vi "Detector GUI.vi"(9 "Standalone":bool=TRUE, 10 "Init Data":variant, 11 "Detector Name":string(combo)="PRIME") -> ()   [LabVIEW 2024]
uses:
  RIMAS Observation Config.ctl
  RIMAS Detector Server Config.ctl
  Detector Class/Detector enum Detector Integration Mode.ctl
  typedefs/CC enum Operation Mode.ctl
  Subsystems/SS typedef cluster Instrument Command Queue Data.ctl
  Subsystems/SS cluster Data Queue type.ctl
  RIMAS Detector Config.ctl
  Detector Class/Detector Image typedef cluster.ctl
  Detector Class/Detector Class.lvclass
  typedefs/CC cluster Observation.ctl
  Observation Queue/CC enum Observation Status.ctl
  Telescope/CC cluster Telescope Offsets.ctl
  typedefs/CC cluster Observation Dither Options.ctl
  typedefs/CC enum Dither Selection.ctl
  Detector Class/Detector cluster Files.ctl
  Detector Class/RIMAS Detector/RIMAS Detector.lvclass
  C:/Development/Prime-RIMAS/Detector/Detector Class/Detector Class.lvclass
  Detector Class/PRIME Detector/PRIME Detector.lvclass
  Detector Simulator/Detector Simulator.lvclass
  typedefs/CC cluster Alarm Data.ctl
  typedefs/CC cluster Exposure.ctl
  Detector Class/Detector Class.lvclass/Detector Class.ctl
  Subsystems/SS cluster New Image Data.ctl
  8cac10b2-9031-4085-930a-abf5b5c9cf51.vi
  Detector Class/Write Object Name.vi
panel:
  in  "Mode":T1
  in  "Tab Control":T2(tab)
  in  "Re-init":bool
  in  "Target Name":string
  out "Number Frames":i32
  in  "Integration Mode":T3
  in  "Integration Time":dbl=3.0 min=3.0 format="%_3g"
  in  "Image List":i32(listbox)
  out "Wait Message":string
  in  "send config":bool
  out "image":sgl[][](graph)
  in  "Get Image":bool
  out "Connected":bool
  in  "Reconnect":bool
  in  "FITS Detector Settings":T4
  in  "Frame Integration Time":dbl
  in  "Sim FITS File Path":path
  in  "Offsets":u16[][](array[numeric]) format="%04x"
  in  "FITS Data File Path":path
  in  "FITS hdr template1":path
  in  "FITS hdr template0":path
  in  "Detector Computer":T5={"Machine"="192.168.121.11", "Password"="", "FITS File Path"="", "Port"=44444, "Header Path"="", "Name"=""}
  in  "Show Log":bool
  in  "Clear Log":bool
  out "Messages":string
  in  "Close":bool
  # "seconds"
  # "Woring 4/8/2022 -- Always force CLOSE when intializing, then \nrestart the server."
  # "sec"
  # "sec"
  # "Seconds"
  # "Use \"Simulation\" if no detector"
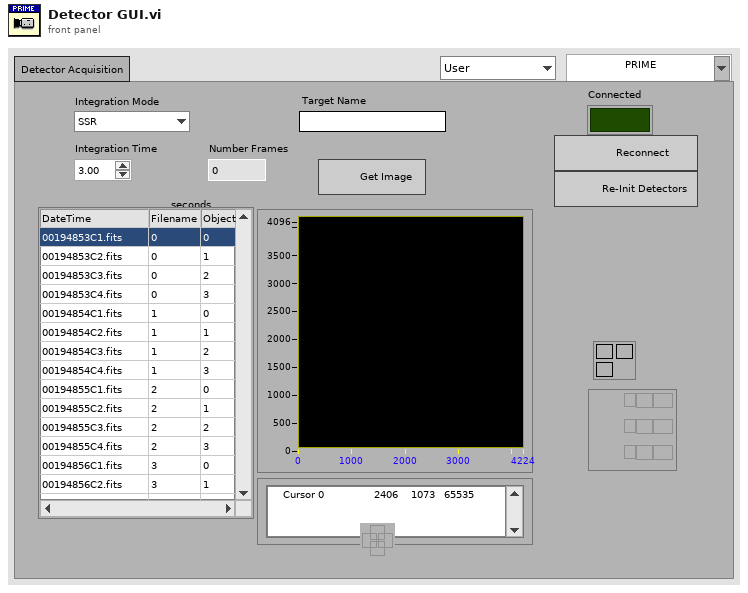
[diagram p1: front panel]
types:
  T1 = typedef "CC enum Operation Mode.ctl" = enum16{"User", "Engineering"}
  T2 = enum32{"Detector Acquisition", "Advanced Settings", "Settings", "Log", "Inputs"}
  T3 = typedef "Detector enum Detector Integration Mode.ctl" = enum16{"SSR", "CDS", "MEAN", "MEDIAN", "MODE", "MIIN", "MAX"}
  T4 = typedef "RIMAS Observation Config.ctl" = cluster{"Exp Time Short":dbl, "# of Frames":dbl, "Exp Time Long":dbl, "# of Groups":dbl, "Object Name":string, "Object":string, "Obs Type":string, "Image Type":string, "Observer":string, "Observer Affiliation":string}
  T5 = typedef "RIMAS Detector Server Config.ctl" = cluster{"Machine":string, "Password":string, "FITS File Path":string, "Port":u16, "Header Path":string, "Name":string}
  T6 = typedef "SS typedef cluster Instrument Command Queue Data.ctl" = cluster{"Cmd":string, "Parameters":variant}
  T7 = typedef "RIMAS Detector Config.ctl" = cluster{"Detector":u16, "Offsets":u16[][], "Detector Computer":T5, "FITS hdr template0":path, "FITS hdr template1":path, "FITS Data File Path":path, "FITS Detector Settings":T4, "Sim Folder":path, "Integration Mode":T3, "Integration Time":dbl, "Frame Int Time":dbl}
  T8 = typedef "Detector Class.lvclass/Detector Image typedef cluster.ctl" = cluster{"Image":sgl[][], "Frame number":i32, "Detector #":u16, "FITS file":path, "File size":i64}
  T9 = typedef "CC cluster Observation.ctl" = cluster{"Priority":i32, "ID":string, "Observer":string, "Obj Name":string, "Obj Type":string, "RA and DEC String":cluster{"RA":string, "DEC":string}, "Filter Wheel 1":string, "Filter Wheel 2":string, "Integration Time":dbl, "Observation Status":T10, "Offsets":T11, "Images":i32, "Dither Options":T12, "Comment 1":string, "Comment 2":string}
  T10 = typedef "CC enum Observation Status.ctl" = enum16{"Ready", "Running", "Done", "Error"}
  T11 = typedef "CC cluster Telescope Offsets.ctl" = cluster{"RA":dbl, "DEC":dbl, "ROT":dbl}
  T12 = typedef "CC cluster Observation Dither Options.ctl" = cluster{"Dither":T13, "Dither Radius":dbl, "Dither Points":i32, "Dither Phase":dbl}
  T13 = typedef "CC enum Dither Selection.ctl" = enum16{"None", "Circle", "Random"}
  T14 = typedef "Detector Class.lvclass/Detector cluster Files.ctl" = cluster{"Time":timestamp, "Files":path[][], "Total Frames":i32}
  T15 = cluster{"state":refnum<user-event>, "cmd q":refnum<queue>, "Cmd":T6, "Data Q":refnum<queue>, "error":errorcluster, "next poll":timestamp, "ch names":string[][], "Detector Config":T7, "images cnt":i32, "Images":T8[], "Name":string, "script q":refnum<queue>, "New Images":T8[], "FITS settings":T4, "Detector ref":refnum<class "Detector Class.lvclass">, "Connected":bool, "Observation":T9, "Raw Files":T14}
  T16 = enum8{"Enabled", "Disabled", "Disabled and Grayed Out"}
  T17 = typedef "CC cluster Alarm Data.ctl" = cluster{"Measured Value":dbl, "Alarm Low":dbl, "Alarm High":dbl, "Message":string, "Source":string}
  T18 = typedef "SS cluster Data Queue type.ctl" = cluster{"Source":string, "Type":string, "Data":variant}
  T19 = typedef "CC cluster Exposure.ctl" = cluster{"Mode":T3, "Integration Time":dbl, "Name":string, "Images":i32}
  T20 = typedef "SS cluster New Image Data.ctl" = cluster{"Frame number":i32, "Detector #":u16, "FITS file":path, "File size":i64}
  T21 = typedef "CC Current Status.ctl" = cluster{"Target":string, "Filter 1":string, "Filter 2":string}
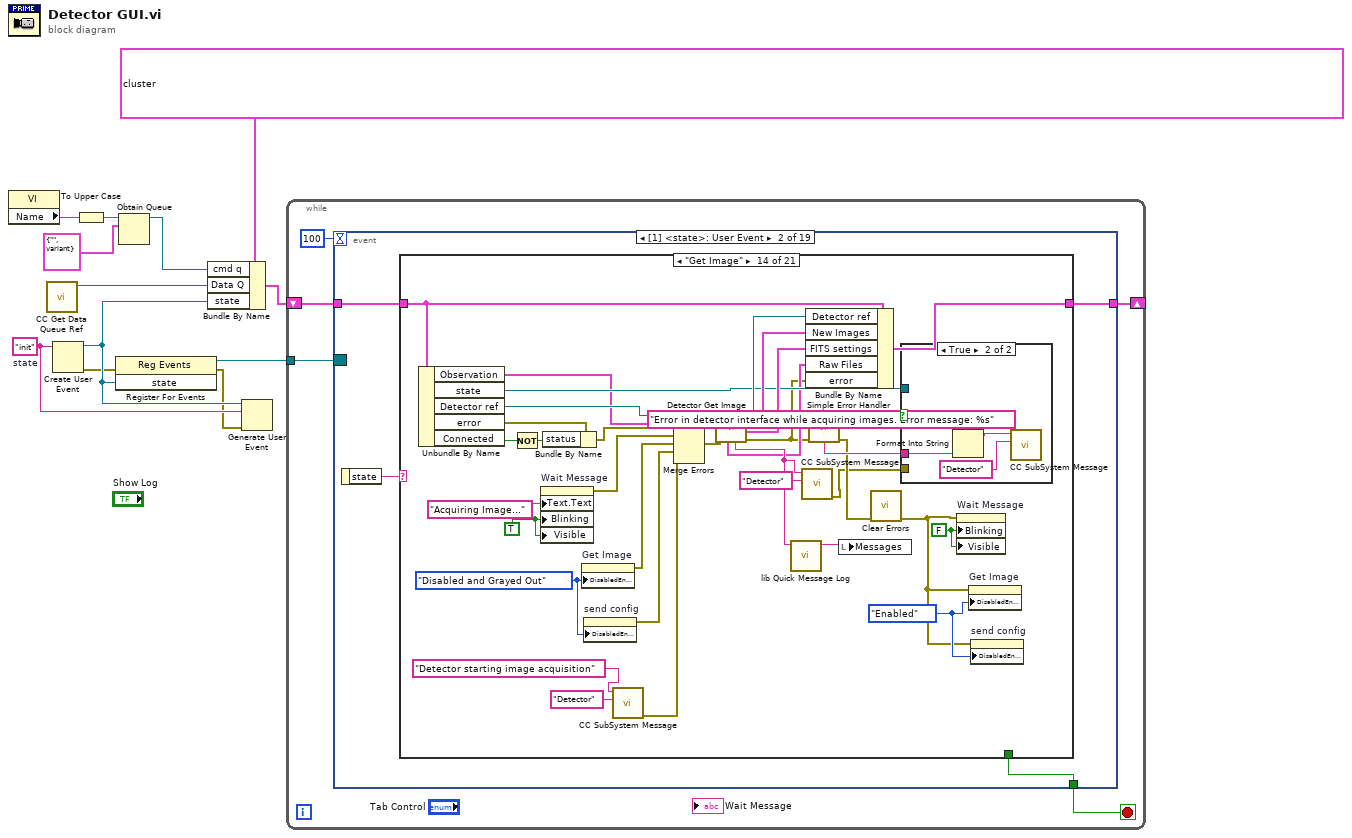
[diagram p0: block diagram]
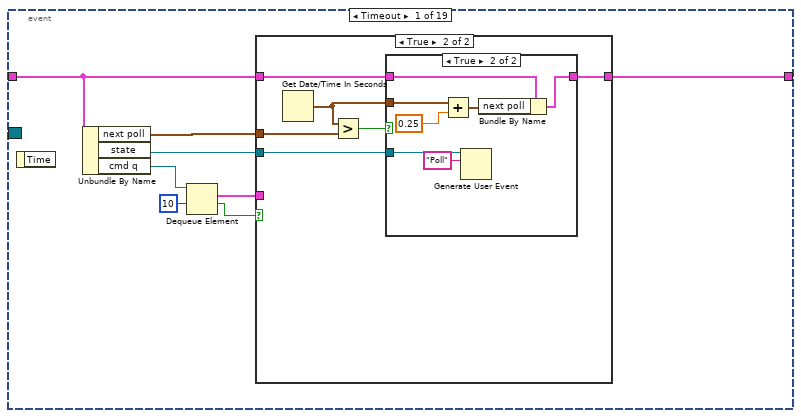
[diagram p2: hidden frame]
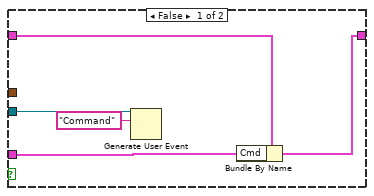
[diagram p3: hidden frame]
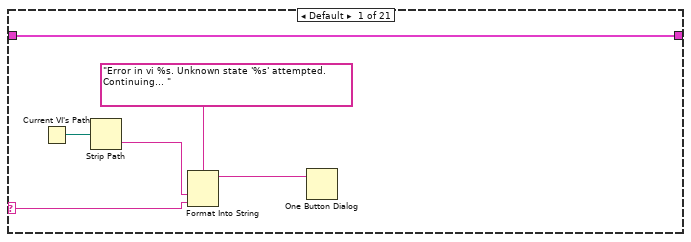
[diagram p5: hidden frame]
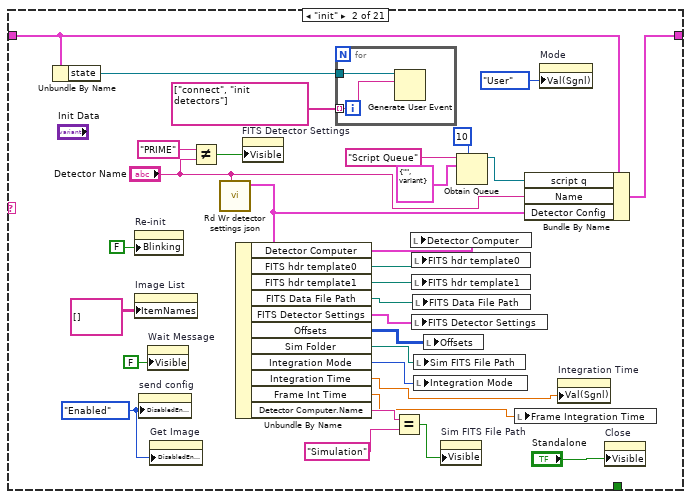
[diagram p6: hidden frame]
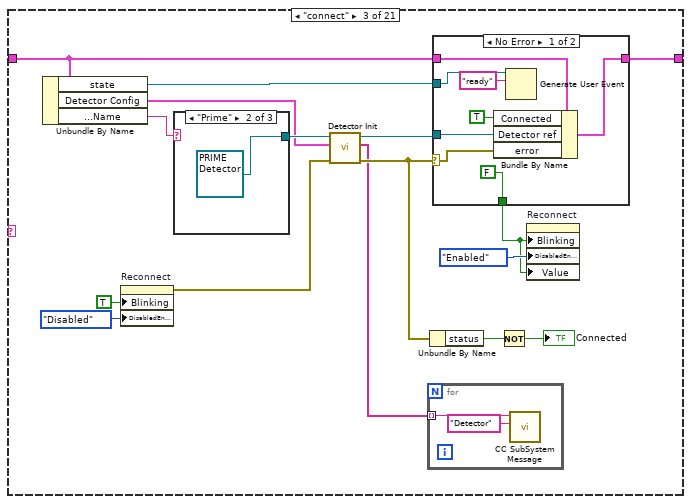
[diagram p7: hidden frame]
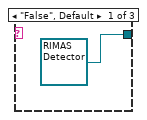
[diagram p8: hidden frame]
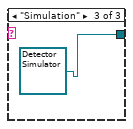
[diagram p9: hidden frame]
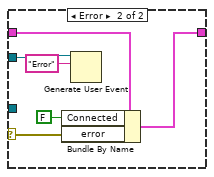
[diagram p10: hidden frame]
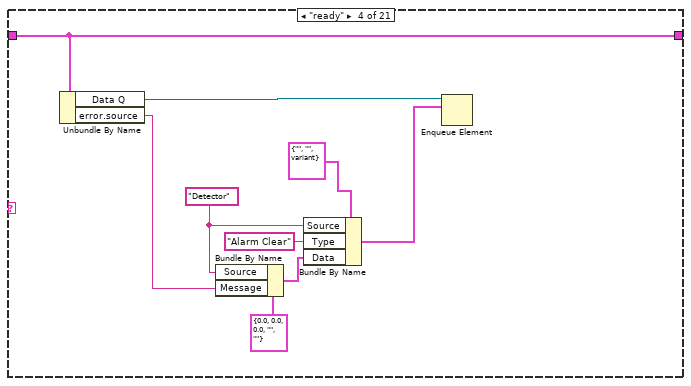
[diagram p11: hidden frame]
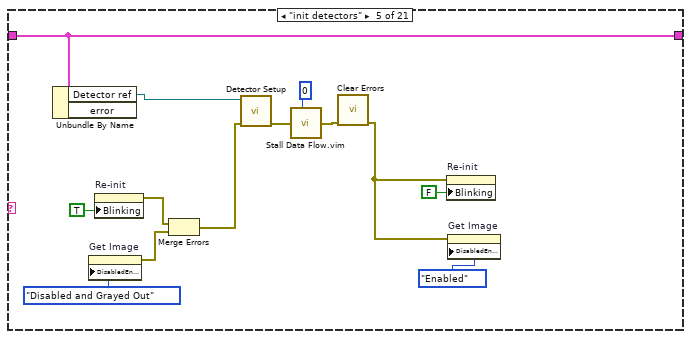
[diagram p12: hidden frame]
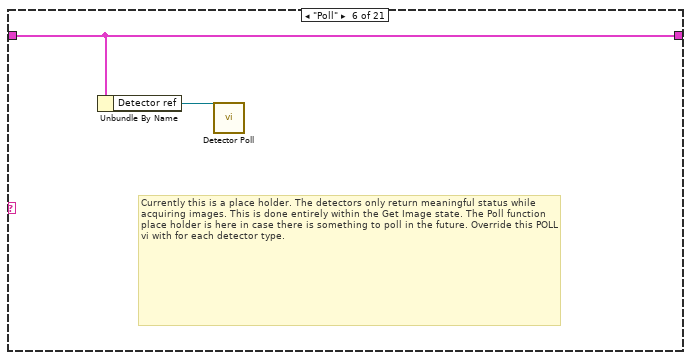
[diagram p13: hidden frame]
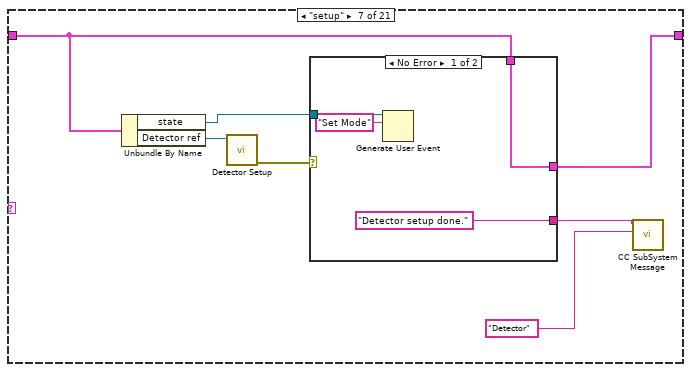
[diagram p14: hidden frame]
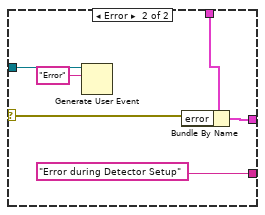
[diagram p15: hidden frame]
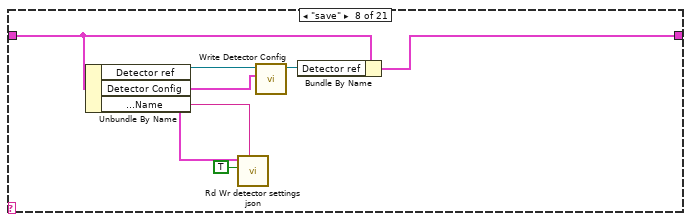
[diagram p16: hidden frame]
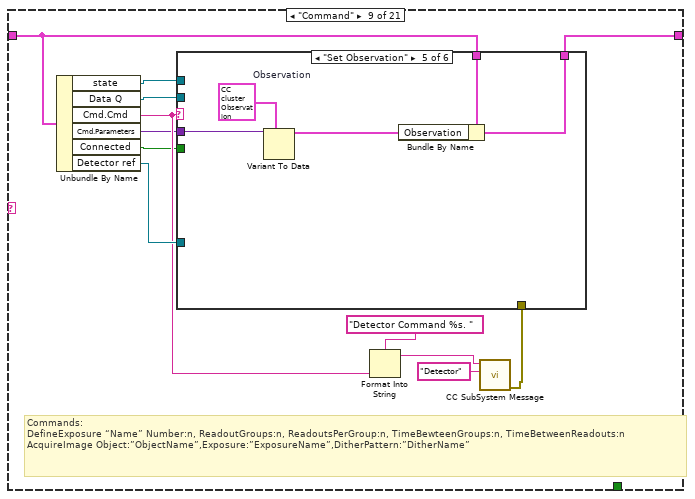
[diagram p17: hidden frame]
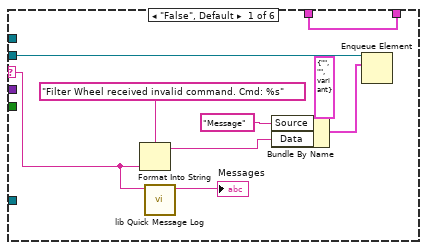
[diagram p18: hidden frame]
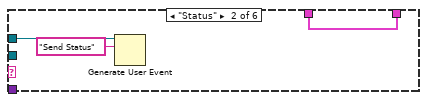
[diagram p19: hidden frame]
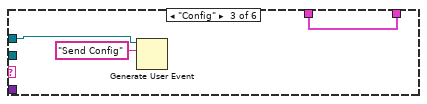
[diagram p20: hidden frame]
diagram:
  w8 = "init"  # state
  n1 = property class="VI"() -> ("Name"=w4:string)  [unwired: 2 in, 2 out]
  n2 = call "CC Get Data Queue Ref.vi"() -> ("Data Q"=w5:refnum<queue>)  [unwired: 10 in, 1 out]
  n3 = Create User Event(user event datatype=w8) -> (user event=w10:refnum<user-event>, error out=w6:errorcluster)  [unwired: 1 in]
  n4 = To Upper Case(1:w4) -> (0:w3:string)
  n5 = register-events(error in=w6, w10) -> (reference out=w9:refnum<event-registration>, error out=w7:errorcluster)  [unwired: 1 in]
  n6 = Obtain Queue(name (unnamed)=w3, element data type=T6 {"Cmd"="", "Parameters"=variant}) -> (queue out=w1:refnum<queue>)  [unwired: 3 in, 2 out]
  n7 = Bundle By Name(cluster=T15 {"state"=refnum, "cmd q"=refnum, "Cmd"={"Cmd"="", "Parameters"=variant}, "Data Q"=refnum, "error"={"status"=FALSE, "code"=0, "source"=""}, "next poll"=timestamp(0 s since 1904-01-01), "ch names"=[], "Detector Config"={"Detector"=0, "Offsets"=[[0, 0, 0, 0, 0, 0, 0, 0, 0, 0, 0, 0, 0, 0, 0, 0, 0, 0, 0, 0, 0, 0, 0, 0, 0, 0, 0, 0, 0, 0, 0, 0]], "Detector Computer"={"Machine"="192.168.121.11", "Password"="", "FITS File Path"="", "Port"=44444, "Header Path"="", "Name"=""}, "FITS hdr template0"=path "", "FITS hdr template1"=path "", "FITS Data File Path"=path "", "FITS Detector Settings"={"Exp Time Short"=0.0, "# of Frames"=0.0, "Exp Time Long"=0.0, "# of Groups"=0.0, "Object Name"="", "Object"="", "Obs Type"="", "Image Type"="", "Observer"="", "Observer Affiliation"=""}, "Sim Folder"=path "", "Integration Mode"=enum."SSR", "Integration Time"=0.0, "Frame Int Time"=0.0}, "images cnt"=0, "Images"=[], "Name"="Simulation", "script q"=refnum, "New Images"=[], "FITS settings"={"Exp Time Short"=0.0, "# of Frames"=0.0, "Exp Time Long"=0.0, "# of Groups"=0.0, "Object Name"="", "Object"="", "Obs Type"="", "Image Type"="", "Observer"="", "Observer Affiliation"=""}, "Detector ref"=refnum, "Connected"=FALSE, "Observation"={"Priority"=0, "ID"="", "Observer"="", "Obj Name"="", "Obj Type"="", "RA and DEC String"={"RA"="HH:MM:SS.nnn", "DEC"="DEG:arcmin:arcsec.nn"}, "Filter Wheel 1"="", "Filter Wheel 2"="", "Integration Time"=0.0, "Observation Status"=enum."Error", "Offsets"={"RA"=0.0, "DEC"=0.0, "ROT"=0.0}, "Images"=0, "Dither Options"={"Dither"=enum."None", "Dither Radius"=0.0, "Dither Points"=0, "Dither Phase"=0.0}, "Comment 1"="", "Comment 2"=""}, "Raw Files"={"Time"=timestamp(0 s since 1904-01-01), "Files"=[], "Total Frames"=0}}, "cmd q"=w1, "Data Q"=w5, "state"=w10) -> (w11:T15)
  n8 = Generate User Event(user event=w10, event data cluster=w8, error in=w7) -> ()  [unwired: 1 in, 2 out]
  n9 = while {
    tunnel: w9 -> [w17]
    shift-right: [w15] -> _
    shift-left: w11 -> [w16]
    stop <- w14 stop-if-true
    n10 = event shown="[1] <state>: User Event" {
      selector: w17 -> [_ _ _ _ _ _ _ _ _ _ _ _ _ _ _ _ _ _ _]
      dyn-events: _ -> [_ _ _ _ _ _ _ _ _ _ _ _ _ _ _ _ _ _ _]
      timeout: 100 -> [_ _ _ _ _ _ _ _ _ _ _ _ _ _ _ _ _ _ _]
      tunnel: w16 -> [w20 w47 w396 w405 w418 w422 w424 w428 w443 w444 w449 w453 w456 w459 w462 w470 w474 w479 w486]
      tunnel: [w19 w46 w396 w405 w415 w422 w424 w429 w443 w444 w449 w453 w456 w460 w465 w473 w477 w482 w486] -> w15
      tunnel: [_ w45 _ _ _ _ _ _ _ _ _ _ _ _ _ _ _ _ _] -> w14
      event Timeout {
        n11 = event-data() -> ()  [unwired: 1 in, 1 out]
        n12 = Unbundle By Name(w20) -> ("next poll"=w18:timestamp, "state"=w21:refnum<user-event>, "cmd q"=w25:refnum<queue>)
        n13 = Dequeue Element(queue=w25, timeout in ms (-1)=10) -> (element=w22:T6, timed out?=w23:bool)  [unwired: 1 in, 2 out]
        n14 = case shown="True" w23 {
          tunnel: w22 -> [w27 _]
          tunnel: w21 -> [w30 w33]
          tunnel: w20 -> [w28 w34]
          tunnel: [w26 w31] -> w19
          tunnel: w18 -> [_ w36]
          frame False {
            n15 = Generate User Event(user event=w30, event data cluster="Command" ("event data")) -> ()  [unwired: 2 in, 2 out]
            n16 = Bundle By Name(cluster=w28, "Cmd"=w27) -> (w26:T15)
          }
          frame True {
            n17 = Get Date/Time In Seconds() -> (seconds since 1Jan1904=w32:timestamp)
            n18 = Greater?(x=w32, y=w36) -> (0:w35:bool)
            n19 = case shown="True" w35 {
              tunnel: w34 -> [w37 w44]
              tunnel: w33 -> [_ w43]
              tunnel: w32 -> [_ w42]
              tunnel: [w37 w39] -> w31
              frame False {
              }
              frame True {
                n20 = Add(x=w42, y=0.25) -> (x+y=w40:timestamp)
                n21 = Generate User Event(user event=w43, event data cluster="Poll" ("event data")) -> ()  [unwired: 2 in, 2 out]
                n22 = Bundle By Name(cluster=w44, "next poll"=w40) -> (w39:T15)
              }
            }
          }
        }
      }
      event User Event {
        n23 = event-data() -> ("state"=w48:string)  [unwired: 1 in]
        n24 = case shown="\"Get Image\"" w48 {
          selector: w48 -> [w53 _ _ _ _ _ _ _ _ _ _ _ _ _ _ _ _ _ _ _ _]
          tunnel: w47 -> [w49 w84 w102 w126 w144 w146 w149 w165 w179 w219 w236 w239 w253 w284 w309 w329 w340 w351 w359 w373 w391]
          tunnel: [w49 w85 w103 w126 w144 w146 w150 w166 w180 w219 w236 w240 w254 w285 w308 w330 w340 w351 w360 w374 w391] -> w46
          tunnel: [_ _ _ _ _ _ _ _ _ _ _ _ _ _ _ _ _ _ _ _ TRUE] -> w45
          frame Default {
            n25 = Current VI's Path() -> (path=w52:path)
            n26 = Strip Path(path=w52) -> (name=w51:string)  [unwired: 1 out]
            n27 = Format Into String(format string="Error in vi %s. Unknown state '%s' attempted. Continuing... ", w51, w53) -> (resulting string=w50:string)  [unwired: 2 in, 1 out]
            n28 = One Button Dialog(message=w50) -> ()  [unwired: 1 in, 1 out]
          }
          frame "init" {
            w71 = T16."Enabled" ("Disabled")
            n29 = Unbundle By Name(w84) -> ("state"=w83:refnum<user-event>)
            n30 = property on="Re-init" class="Bool"("Blinking"=FALSE) -> ()  [unwired: 2 in, 2 out]
            n31 = property on="Image List" class="MCListbox (strict)"("ItemNames"=string[][] [] ("Item Names")) -> ()  [unwired: 2 in, 2 out]
            n32 = property on="send config" class="Bool"("DisabledEnum"=w71) -> ()  [unwired: 2 in, 2 out]
            n33 = property on="Wait Message" class="Str"("Visible"=FALSE) -> ()  [unwired: 2 in, 2 out]
            n34 = property on="Get Image" class="Bool"("DisabledEnum"=w71) -> ()  [unwired: 2 in, 2 out]
            n35 = Not Equal?(x="PRIME", y="Detector Name") -> (x != y?=w58:bool)
            n36 = call "Rd Wr detector settings json.vi"("Detector Name"="Detector Name") -> ("Detector Config"=w80:T7)  [unwired: 9 in, 1 out]
            n37 = Unbundle By Name(w80) -> ("Detector Computer"=w79:T5, "FITS hdr template0"=w78:path, "FITS hdr template1"=w77:path, "FITS Data File Path"=w76:path, "FITS Detector Settings"=w75:T4, "Offsets"=w74:u16[][], "Sim Folder"=w73:path, "Integration Mode"=w62:T3, "Integration Time"=w61:dbl, "Frame Int Time"=w57:dbl, "Detector Computer.Name"=w70:string)
            n38 = property on="FITS Detector Settings" class="Clust (strict)"("Visible"=w58) -> ()  [unwired: 2 in, 2 out]
            n39 = for {
              tunnel: w83 -> [w87]
              tunnel: string[] ["connect", "init detectors"] -> [w86] mode=indexing
              n40 = Generate User Event(user event=w87, event data cluster=w86) -> ()  [unwired: 2 in, 2 out]
            }
            n41 = Equal?(x=w70, y="Simulation") -> (x = y?=w68:bool)
            n42 = local write "Detector Computer"(w79) -> ()
            n43 = local write "FITS hdr template0"(w78) -> ()
            n44 = local write "FITS hdr template1"(w77) -> ()
            n45 = local write "FITS Detector Settings"(w75) -> ()
            n46 = local write "FITS Data File Path"(w76) -> ()
            n47 = local write "Sim FITS File Path"(w73) -> ()
            n48 = local write "Integration Mode"(w62) -> ()
            n49 = local write "Offsets"(w74) -> ()
            n50 = property on="Sim FITS File Path" class="Path"("Visible"=w68) -> ()  [unwired: 2 in, 2 out]
            n51 = Obtain Queue(max queue size (-1, unlimited)=10, name (unnamed)="Script Queue", element data type=T6 {"Cmd"="", "Parameters"=variant}) -> (queue out=w63:refnum<queue>)  [unwired: 2 in, 2 out]
            n52 = local write "Frame Integration Time"(w57) -> ()
            n53 = Bundle By Name(cluster=w84, "script q"=w63, "Name"="Detector Name", "Detector Config"=w80) -> (w85:T15)
            n54 = property on="Mode" class="Enum (strict)"("Val(Sgnl)"=CC_enum_Operation_Mode."User" ("Value (Signaling)")) -> ()  [unwired: 2 in, 2 out]
            n55 = property on="Integration Time" class="DigNum (strict)"("Val(Sgnl)"=w61) -> ()  [unwired: 2 in, 2 out]
            n56 = property on="Close" class="Bool"("Visible"="Standalone") -> ()  [unwired: 2 in, 2 out]
          }
          frame "connect" {
            n57 = Unbundle By Name(w102) -> ("state"=w101:refnum<user-event>, "Detector Config"=w93:T7, "Detector Config.Detector Computer.Name"=w98:string)
            n58 = property on="Reconnect" class="Bool (strict)"("Blinking"=TRUE, "DisabledEnum"=T16."Disabled" ("Disabled")) -> (error out=w90:errorcluster)  [unwired: 2 in, 1 out]
            n59 = case shown="\"Prime\"" w98 {
              tunnel: [refnum<class "RIMAS Detector.lvclass"> refnum ("RIMAS Detector.lvclass") refnum<class "PRIME Detector.lvclass"> refnum ("PRIME Detector.lvclass") refnum<class "Detector Simulator.lvclass"> refnum ("Detector Simulator.lvclass")] -> w97
              frame "False", Default {
              }
              frame "Prime" {
              }
              frame "Simulation" {
              }
            }
            n60 = call-dynamic "Detector Init.vi"("error in (no error)"=w90, "Detector Config"=w93, "Detector Class in"=w97) -> ("error out"=w95:errorcluster, "Log Messages"=w94:string[], "Detector Class out"=w96:refnum<class "Detector Class.lvclass">)  [unwired: 6 in]
            n61 = for {
              tunnel: w94 -> [w105] mode=indexing
              n62 = call "CC SubSystem Message.vi"("Subsystem"="Detector", "Message"=w105) -> ()  [unwired: 9 in, 1 out]
            }
            n63 = Unbundle By Name(w95) -> ("status"=w100:bool)
            n64 = case shown="No Error" w95 {
              selector: w95 -> [w109 w122]
              tunnel: w96 -> [w116 _]
              tunnel: [w115 w121] -> w103
              tunnel: w102 -> [w114 w120]
              tunnel: w101 -> [w111 w119]
              tunnel: [FALSE ("Blinking") _] -> w88
              frame No Error {
                n65 = Bundle By Name(cluster=w114, "Connected"=TRUE, "Detector ref"=w116, "error"=w109) -> (w115:T15)
                n66 = Generate User Event(user event=w111, event data cluster="ready" ("event data")) -> ()  [unwired: 2 in, 2 out]
              }
              frame Error {
                n67 = Bundle By Name(cluster=w120, "Connected"=FALSE, "error"=w122) -> (w121:T15)
                n68 = Generate User Event(user event=w119, event data cluster="Error" ("event data")) -> ()  [unwired: 2 in, 2 out]
              }
            }
            n69 = Not(x=w100) -> (.not. x?=→"Connected":bool)
            n70 = property on="Reconnect" class="Bool (strict)"("Blinking"=w88, "DisabledEnum"=T16."Enabled" ("Disabled"), "Value"=w88) -> ()  [unwired: 2 in, 2 out]
          }
          frame "ready" {
            w124 = "Detector" ("Source")
            n71 = Unbundle By Name(w126) -> ("Data Q"=w125:refnum<queue>, "error.source"=w123:string)
            n72 = Bundle By Name(cluster=T17 {"Measured Value"=0.0, "Alarm Low"=0.0, "Alarm High"=0.0, "Message"="", "Source"=""} ("element"), "Source"=w124, "Message"=w123) -> (w127:T17)
            n73 = Bundle By Name(cluster=T18 {"Source"="", "Type"="", "Data"=variant} ("element"), "Source"=w124, "Type"="Alarm Clear", "Data"=w127) -> (w129:T18)
            n74 = Enqueue Element(queue=w125, element=w129) -> ()  [unwired: 2 in, 3 out]
          }
          frame "init detectors" {
            n75 = Unbundle By Name(w144) -> ("Detector ref"=w143:refnum<class "Detector Class.lvclass">)  [unwired: 1 out]
            n76 = property on="Get Image" class="Bool"("DisabledEnum"=T16."Disabled and Grayed Out" ("Disabled")) -> (error out=w138:errorcluster)  [unwired: 2 in, 1 out]
            n77 = property on="Re-init" class="Bool"("Blinking"=TRUE) -> (error out=w140:errorcluster)  [unwired: 2 in, 1 out]
            n78 = Merge Errors(w140, w138) -> (w139:errorcluster)
            n79 = call-dynamic "Detector Setup.vi"("error in (no error)"=w139, "Detector Class in"=w143) -> ("error out"=w134:errorcluster)  [unwired: 7 in, 2 out]
            n80 = call "Stall Data Flow.vim"("value in"=w134, "milliseconds to wait"=u32 0) -> ("value out"=w133:errorcluster)  [unwired: 1 out]
            n81 = call <vilib>:"Clear Errors.vi"("error in (no error)"=w133) -> ("error out"=w135:errorcluster)  [unwired: 5 in, 1 out]
            n82 = property on="Re-init" class="Bool"(error in=w135, "Blinking"=FALSE) -> ()  [unwired: 1 in, 2 out]
            n83 = property on="Get Image" class="Bool"(error in=w135, "DisabledEnum"=T16."Enabled" ("Disabled")) -> ()  [unwired: 1 in, 2 out]
          }
          frame "Poll" {
            # "Currently this is a place holder. The detectors only return meaningful status while acquiring images. This is done entirely within the Get Image state. The Poll function place holder is here in case there is something to poll in the future. Override this POLL vi with for each detector type."
            n84 = Unbundle By Name(w146) -> ("Detector ref"=w145:refnum<class "Detector Class.lvclass">)
            n85 = call-dynamic "Detector Poll.vi"("Detector Class in"=w145) -> ()  [unwired: 8 in, 3 out]
          }
          frame "setup" {
            n86 = Unbundle By Name(w149) -> ("state"=w151:refnum<user-event>, "Detector ref"=w153:refnum<class "Detector Class.lvclass">)
            n87 = call-dynamic "Detector Setup.vi"("Detector Class in"=w153) -> ("error out"=w152:errorcluster)  [unwired: 8 in, 2 out]
            n88 = case shown="No Error" w152 {
              selector: w152 -> [_ w160]
              tunnel: w151 -> [w155 w163]
              tunnel: w149 -> [w157 w161]
              tunnel: [w157 w159] -> w150
              tunnel: ["Detector setup done." "Error during Detector Setup"] -> w147
              frame No Error {
                n89 = Generate User Event(user event=w155, event data cluster="Set Mode" ("event data")) -> ()  [unwired: 2 in, 2 out]
              }
              frame Error {
                n90 = Generate User Event(user event=w163, event data cluster="Error" ("event data")) -> ()  [unwired: 2 in, 2 out]
                n91 = Bundle By Name(cluster=w161, "error"=w160) -> (w159:T15)
              }
            }
            n92 = call "CC SubSystem Message.vi"("Subsystem"="Detector", "Message"=w147) -> ()  [unwired: 9 in, 1 out]
          }
          frame "save" {
            n93 = Unbundle By Name(w165) -> ("Detector ref"=w169:refnum<class "Detector Class.lvclass">, "Detector Config"=w168:T7, "Detector Config.Detector Computer.Name"=w164:string)
            n94 = call "Rd Wr detector settings json.vi"("Detector Name"=w164, "Write? (F:Read)"=TRUE, "Detector Config"=w168) -> ()  [unwired: 7 in, 2 out]
            n95 = call-dynamic "Write Detector Config.vi"("Detector Config"=w168, "Detector Class in"=w169) -> ("Detector Class out"=w167:refnum<class "Detector Class.lvclass">)  [unwired: 8 in, 1 out]
            n96 = Bundle By Name(cluster=w165, "Detector ref"=w167) -> (w166:T15)
          }
          frame "Command" {
            # "Commands:\nDefineExposure “Name” Number:n, ReadoutGroups:n, ReadoutsPerGroup:n, TimeBewteenGroups:n, TimeBetweenReadouts:n\nAcquireImage Object:”ObjectName”,Exposure:”ExposureName”,DitherPattern:”DitherName”"
            n97 = Unbundle By Name(w179) -> ("state"=w181:refnum<user-event>, "Data Q"=w182:refnum<queue>, "Cmd.Cmd"=w176:string, "Cmd.Parameters"=w175:variant, "Connected"=w174:bool, "Detector ref"=w178:refnum<class "Detector Class.lvclass">)
            n98 = Format Into String(format string="Detector Command %s. ", w176) -> (resulting string=w171:string)  [unwired: 2 in, 1 out]
            n99 = call "CC SubSystem Message.vi"("Subsystem"="Detector", "Message"=w171) -> ("error out"=w172:errorcluster)  [unwired: 9 in]
            n100 = case shown="\"Set Observation\"" w176 {
              selector: w176 -> [w185 _ _ _ _ _]
              tunnel: w182 -> [w191 _ _ _ _ _]
              tunnel: w175 -> [_ _ _ _ w211 _]
              tunnel: w181 -> [_ w194 w196 w200 _ w214]
              tunnel: w179 -> [w183 w192 w195 w199 w209 w212]
              tunnel: [w183 w192 w195 w199 w208 w212] -> w180
              tunnel: w178 -> [_ _ _ _ _ _]
              tunnel: w174 -> [_ _ _ w198 _ _]
              tunnel: w172 -> [_ _ _ _ _ _]
              frame "False", Default {
                n101 = Format Into String(format string="Filter Wheel received invalid command. Cmd: %s", w185) -> (resulting string=w187:string)  [unwired: 2 in, 1 out]
                n102 = call "lib Quick Message Log.vi"("Message"=w185) -> ("Log"=→"Messages":string)  [unwired: 9 in, 1 out]
                n103 = Bundle By Name(cluster=T18 {"Source"="", "Type"="", "Data"=variant} ("element"), "Source"="Message" ("Data Type"), "Data"=w187) -> (w186:T18)
                n104 = Enqueue Element(queue=w191, element=w186) -> ()  [unwired: 2 in, 3 out]
              }
              frame "Status" {
                n105 = Generate User Event(user event=w194, event data cluster="Send Status" ("event data")) -> ()  [unwired: 2 in, 2 out]
              }
              frame "Config" {
                n106 = Generate User Event(user event=w196, event data cluster="Send Config" ("event data")) -> ()  [unwired: 2 in, 2 out]
              }
              frame "Acquire Image" {
                n107 = case shown="False" w198 {
                  tunnel: w200 -> [w204 w206]
                  frame False {
                    n108 = Generate User Event(user event=w204, event data cluster="image acq error" ("event data")) -> ()  [unwired: 2 in, 2 out]
                    n109 = call "CC SubSystem Message.vi"("Subsystem"="Detector", "Message"="Detector not responding. Cannot acquire images." ("format string")) -> ()  [unwired: 9 in, 1 out]
                  }
                  frame True {
                    n110 = Generate User Event(user event=w206, event data cluster="Acquire Image" ("event data")) -> ()  [unwired: 2 in, 2 out]
                  }
                }
              }
              frame "Set Observation" {
                w210 = T9 {"Priority"=0, "ID"="", "Observer"="", "Obj Name"="", "Obj Type"="", "RA and DEC String"={"RA"="HH:MM:SS.nnn", "DEC"="DEG:arcmin:arcsec.nn"}, "Filter Wheel 1"="", "Filter Wheel 2"="", "Integration Time"=0.0, "Observation Status"=enum."Error", "Offsets"={"RA"=0.0, "DEC"=0.0, "ROT"=0.0}, "Images"=0, "Dither Options"={"Dither"=enum."None", "Dither Radius"=0.0, "Dither Points"=0, "Dither Phase"=0.0}, "Comment 1"="", "Comment 2"=""}  # Observation
                n111 = Variant To Data(type=w210, Variant=w211) -> (data=w207:T9)  [unwired: 1 in, 1 out]
                n112 = Bundle By Name(cluster=w209, "Observation"=w207) -> (w208:T15)
              }
              frame "Shutdown" {
                n113 = Generate User Event(user event=w214, event data cluster="Shutdown" ("event data")) -> ()  [unwired: 2 in, 2 out]
              }
            }
          }
          frame "Send Status" {
            n114 = Unbundle By Name(w219) -> ("Data Q"=w218:refnum<queue>)
            n115 = Bundle By Name(cluster=T18 {"Source"="", "Type"="", "Data"=variant} ("element"), "Source"="Detector" ("Data Type")) -> (w215:T18)
            n116 = Enqueue Element(queue=w218, element=w215) -> ()  [unwired: 2 in, 3 out]
          }
          frame "Error" {
            w224 = "Detector" ("Source")
            n117 = Unbundle By Name(w236) -> ("error"=w235:errorcluster, "Data Q"=w222:refnum<queue>)
            n118 = call <vilib>:"Simple Error Handler.vi"("error in (no error)"=w235) -> ("source out"=w223:string, "message"=w230:string)  [unwired: 4 in, 3 out]
            n119 = local read "Messages"() -> (w234:string)
            n120 = Bundle By Name(cluster=T17 {"Measured Value"=0.0, "Alarm Low"=0.0, "Alarm High"=0.0, "Message"="", "Source"=""} ("element"), "Source"=w224, "Message"=w223) -> (w225:T17)
            n121 = Concatenate Strings(w234, "\r\n", w230) -> (w232:string)
            n122 = Format Into String(format string="Detector Error Message: \"%s\"", w230) -> (resulting string=w220:string)  [unwired: 2 in, 1 out]
            n123 = Bundle By Name(cluster=T18 {"Source"="", "Type"="", "Data"=variant} ("element"), "Source"=w224, "Type"="Alarm Set", "Data"=w225) -> (w227:T18)
            n124 = local write "Messages"(w232) -> ()
            n125 = Enqueue Element(queue=w222, element=w227) -> ()  [unwired: 2 in, 3 out]
            n126 = call "CC SubSystem Message.vi"("Subsystem"="Detector", "Message"=w220) -> ()  [unwired: 9 in, 1 out]
          }
          frame "Set Mode" {
            n127 = Unbundle By Name(w239) -> ("Detector ref"=w242:refnum<class "Detector Class.lvclass">)
            n128 = call-dynamic "Detector Set Config.vi"("Detector Class in"=w242) -> ("Detector Class out"=w241:refnum<class "Detector Class.lvclass">)  [unwired: 9 in, 1 out]
            n129 = Bundle By Name(cluster=w239, "Detector ref"=w241) -> (w240:T15)
            n130 = call "CC SubSystem Message.vi"("Subsystem"="Detector", "Message"="Detector Mode Set") -> ()  [unwired: 9 in, 1 out]
          }
          frame "Acquire Image" {
            n131 = Unbundle By Name(w253) -> ("state"=w252:refnum<user-event>, "Cmd.Parameters"=w256:variant, "Detector ref"=w255:refnum<class "Detector Class.lvclass">)
            n132 = call "Rd Wr Current Status json.vi"() -> ("Current Status"=w258:T21)  [unwired: 10 in, 1 out]
            n133 = Unbundle By Name(w258) -> ("Target"=w257:string)
            n134 = property class="Detector Class.lvclass"(reference=w255, "Object Name"=w257) -> (reference out=w249:refnum<class "Detector Class.lvclass">)  [unwired: 1 in, 1 out]
            n135 = Variant To Data(type=T19 {"Mode"=enum."CDS", "Integration Time"=1.0, "Name"="", "Images"=1} ("Exposure in"), Variant=w256) -> (data=w260:T19)  [unwired: 1 in, 1 out]
            n136 = local write "Target Name"(w257) -> ()
            n137 = Generate User Event(user event=w252, event data cluster="Get Image" ("event data")) -> ()  [unwired: 2 in, 2 out]
            n138 = Unbundle By Name(w260) -> ("Integration Time"=w243:dbl, "Name"=w244:string)
            n139 = call-dynamic "Read Detector Config.vi"("Detector Class in"=w249) -> ("Detector Config"=w247:T7, "Detector Class out"=w248:refnum<class "Detector Class.lvclass">)  [unwired: 8 in, 1 out]
            n140 = Bundle By Name(cluster=w247, "Integration Mode"=Detector_enum_Detector_Integration_Mode."CDS" ("Detector Config.Integration Mode"), "Integration Time"=w243) -> (w246:T7)
            n141 = call-dynamic "Write Detector Config.vi"("Detector Config"=w246, "Detector Class in"=w248) -> ("Detector Class out"=w250:refnum<class "Detector Class.lvclass">)  [unwired: 8 in, 1 out]
            n142 = Bundle By Name(cluster=w253, "Detector Config.Integration Mode"=Detector_enum_Detector_Integration_Mode."CDS", "Detector Config.Integration Time"=w243, "Detector Config.FITS Detector Settings.Object Name"=w244, "Detector ref"=w250) -> (w254:T15)
          }
          frame "Get Image" {
            (unwired) "Erri" ("message")
            w291 = TRUE ("Blinking")
            w292 = FALSE ("Blinking")
            w293 = T16."Enabled" ("Disabled")
            w294 = T16."Disabled and Grayed Out" ("Disabled")
            n143 = Unbundle By Name(w284) -> ("Observation"=w262:T9, "state"=w275:refnum<user-event>, "Detector ref"=w295:refnum<class "Detector Class.lvclass">, "error"=w274:errorcluster, "Connected"=w273:bool)
            n144 = Not(x=w273) -> (.not. x?=w271:bool)
            n145 = property on="Wait Message" class="Str"("Text.Text"="Acquiring Image...", "Blinking"=w291, "Visible"=w291) -> (error out=w289:errorcluster)  [unwired: 2 in, 1 out]
            n146 = Bundle By Name(cluster=w274, "status"=w271) -> (w272:errorcluster)
            n147 = property on="Get Image" class="Bool"("DisabledEnum"=w294) -> (error out=w288:errorcluster)  [unwired: 2 in, 1 out]
            n148 = property on="send config" class="Bool"("DisabledEnum"=w294) -> (error out=w287:errorcluster)  [unwired: 2 in, 1 out]
            n149 = call "CC SubSystem Message.vi"("Subsystem"="Detector", "Message"="Detector starting image acquisition") -> ("error out"=w265:errorcluster)  [unwired: 9 in]
            n150 = Merge Errors(w272, w289, w288, w287, w265) -> (w286:errorcluster)
            n151 = call-dynamic "Detector Get Image.vi"("error in (no error)"=w286, "Observation"=w262, "Detector Class in"=w295) -> ("error out"=w263:errorcluster, "FITS Detector Settings"=w277:T4, "Images"=w278:T8[], "Detector Class out"=w279:refnum<class "Detector Class.lvclass">, "Message Log"=w269:string, "Detector Files"=w264:T14)  [unwired: 3 in]
            n152 = call "lib Quick Message Log.vi"("Message"=w269) -> ("Log"=w276:string)  [unwired: 9 in, 1 out]
            n153 = call "CC SubSystem Message.vi"("Subsystem"="Detector", "Message"=w269) -> ("error out"=w268:errorcluster)  [unwired: 9 in]
            n154 = Bundle By Name(cluster=w284, "Detector ref"=w279, "New Images"=w278, "FITS settings"=w277, "Raw Files"=w264, "error"=w263) -> (w285:T15)
            n155 = call <vilib>:"Simple Error Handler.vi"("error in (no error)"=w263) -> ("error?"=w283:bool, "error out"=w280:errorcluster, "message"=w282:string)  [unwired: 4 in, 2 out]
            n156 = local write "Messages"(w276) -> ()
            n157 = call <vilib>:"Clear Errors.vi"("error in (no error)"=w280) -> ("error out"=w281:errorcluster)  [unwired: 5 in, 1 out]
            n158 = case shown="True" w283 {
              tunnel: w282 -> [_ w300]
              tunnel: w268 -> [_ _]
              tunnel: w275 -> [w297 _]
              frame False {
                n159 = Generate User Event(user event=w297, event data cluster="Process Images" ("event data")) -> ()  [unwired: 2 in, 2 out]
              }
              frame True {
                n160 = Format Into String(format string="Error in detector interface while acquiring images. Error message: %s", w300) -> (resulting string=w298:string)  [unwired: 2 in, 1 out]
                n161 = call "CC SubSystem Message.vi"("Subsystem"="Detector", "Message"=w298) -> ()  [unwired: 9 in, 1 out]
              }
            }
            n162 = property on="Wait Message" class="Str"(error in=w281, "Blinking"=w292, "Visible"=w292) -> ()  [unwired: 1 in, 2 out]
            n163 = property on="Get Image" class="Bool"(error in=w281, "DisabledEnum"=w293) -> ()  [unwired: 1 in, 2 out]
            n164 = property on="send config" class="Bool"(error in=w281, "DisabledEnum"=w293) -> ()  [unwired: 1 in, 2 out]
          }
          frame "Process Images" {
            n165 = Unbundle By Name(w309) -> ("Observation"=w305:T9, "New Images"=w313:T8[], "Detector Config"=w312:T7, "Raw Files"=w311:T14)
            n166 = call "Detector Process Images.vi"("Observation"=w305, "Raw Files"=w311, "Detector Config"=w312, "Images"=w313) -> ("Table"=w303:string[], "Images out"=w310:T8[])  [unwired: 5 in, 1 out]
            n167 = Build Array(w303) -> (w302:string[][])
            n168 = Bundle By Name(cluster=w309, "New Images"=w310) -> (w308:T15)
            n169 = disable-structure shown="Disabled" {
              disable-tunnel: string[] ["DateTime", "Filename", "Object", "Filter1", "Filter2", "Chip", "NFrames", "Frame", "Nint", "Int", "ExpTime"] ("Header") -> [w315 _]
              disable-tunnel: w302 -> [w314 _]
              frame Disabled {
                n170 = property on="Image List" class="MCListbox (strict)"("ItemNames"=w314, "ColHdrString"=w315) -> ()  [unwired: 2 in, 2 out]
              }
              frame Enabled {
              }
            }
            n171 = Unbundle By Name(w308) -> ("state"=w307:refnum<user-event>)
            n172 = Generate User Event(user event=w307, event data cluster="Add Images" ("event data")) -> ()  [unwired: 2 in, 2 out]
          }
          frame "Add Images" {
            # "Send info but not image data in queue"
            n173 = Unbundle By Name(w329) -> ("state"=w327:refnum<user-event>, "New Images"=w317:T8[], "script q"=w324:refnum<queue>, "Data Q"=w323:refnum<queue>)  [unwired: 2 out]
            n174 = call "Detector Send New Image Message.vi"("New Images"=w317) -> ("Image Messages"=w320:T20[])  [unwired: 9 in, 1 out]
            n175 = disable-structure shown="Enabled" {
              disable-tunnel: "Update Image List" ("event data") -> [w337 _]
              disable-tunnel: w327 -> [w336 _]
              frame Enabled {
                n176 = Generate User Event(user event=w336, event data cluster=w337) -> ()  [unwired: 2 in, 2 out]
              }
              frame Disabled {
              }
            }
            n177 = local read "Image List"() -> (w334:i32)
            n178 = Bundle By Name(cluster=T6 {"Cmd"="New Images", "Parameters"=variant} ("element"), "Parameters"=w320) -> (w322:T6)
            n179 = Bundle By Name(cluster=T18 {"Source"="Detector", "Type"="New Image", "Data"=variant} ("element"), "Data"=w320) -> (w319:T18)
            n180 = Index Array(array=w317, index=w334) -> (element=w335:T8)
            n181 = Array Size(array=w317) -> (size(s)=w326:i32)
            n182 = Unbundle By Name(w335) -> ("Image"=→"image":sgl[][])
            n183 = Decrement(x=w326) -> (x-1=w325:i32)
            n184 = Bundle By Name(cluster=w329, "Images"=w317) -> (w330:T15)
            n185 = call "Detector Send Data to Data Q.vi"("element"=w319, "Data Q"=w323) -> ("error out"=w318:errorcluster)  [unwired: 9 in]
            n186 = Enqueue Element(queue=w324, element=w322, timeout in ms (-1)=0) -> (error out=w331:errorcluster)  [unwired: 1 in, 2 out]
            n187 = call <vilib>:"Clear Errors.vi"("error in (no error)"=w331) -> ()  [unwired: 5 in, 2 out]
            n188 = property on="Image List" class="MCListbox (strict)"("Val(Sgnl)"=w325) -> ()  [unwired: 2 in, 2 out]
            n189 = call <vilib>:"Clear Errors.vi"("error in (no error)"=w318) -> ()  [unwired: 5 in, 2 out]
          }
          frame "Update Image List" {
            n190 = Unbundle By Name(w340) -> ("Images"=w339:T8[])
            n191 = for {
              tunnel: w339 -> [w348] mode=indexing
              tunnel: [w343] -> w338 mode=indexing
              n192 = Unbundle By Name(w348) -> ("FITS file"=w342:path, "Detector #"=w347:u16, "Frame number"=w346:i32)
              n193 = Number To Decimal String(number=w347) -> (decimal integer string=w344:string)  [unwired: 1 in]
              n194 = Strip Path(path=w342) -> (name=w341:string)  [unwired: 1 out]
              n195 = Number To Decimal String(number=w346) -> (decimal integer string=w345:string)  [unwired: 1 in]
              n196 = Build Array(w341, w344, w345) -> (w343:string[])
            }
            n197 = property on="Image List" class="MCListbox (strict)"("ItemNames"=w338) -> ()  [unwired: 2 in, 2 out]
          }
          frame "image acq error" {
            # "send empty array of images to tell script to contunie"
            n198 = Unbundle By Name(w351) -> ("script q"=w350:refnum<queue>)
            n199 = Bundle By Name(cluster=T6 {"Cmd"="New Images", "Parameters"=variant} ("element"), "Parameters"=T20[] [] ("Image Messages")) -> (w352:T6)
            n200 = Enqueue Element(queue=w350, element=w352, timeout in ms (-1)=0) -> (error out=w353:errorcluster)  [unwired: 1 in, 2 out]
            n201 = call <vilib>:"Clear Errors.vi"("error in (no error)"=w353) -> ()  [unwired: 5 in, 2 out]
          }
          frame "Configure" {
            n202 = Unbundle By Name(w359) -> ("Detector ref"=w362:refnum<class "Detector Class.lvclass">, "Detector Config"=w358:T7)
            n203 = call-dynamic "Write Detector Config.vi"("Detector Config"=w358, "Detector Class in"=w362) -> ("Detector Class out"=w361:refnum<class "Detector Class.lvclass">)  [unwired: 8 in, 1 out]
            n204 = Bundle By Name(cluster=w359, "Detector ref"=w361) -> (w360:T15)
            n205 = call "CC SubSystem Message.vi"("Subsystem"="Detector", "Message"="Detector Configure") -> ()  [unwired: 9 in, 1 out]
          }
          frame "Send FITS Files" {
            w365 = FALSE ("Blinking")
            w366 = TRUE ("Blinking")
            n206 = Unbundle By Name(w373) -> ("Detector ref"=w371:refnum<class "Detector Class.lvclass">)
            n207 = property on="Wait Message" class="Str"("Text.Text"="Sending Header to Detector", "Blinking"=w366, "Visible"=w366) -> (error out=w369:errorcluster)  [unwired: 2 in, 1 out]
            n208 = call-dynamic "Detector Make FITS Templates.vi"("error in (no error)"=w369, "Detector Class in"=w371) -> ("error out"=w368:errorcluster)  [unwired: 8 in, 1 out]
            n209 = Unbundle By Name(w373) -> ("state"=w375:refnum<user-event>)
            n210 = property on="Wait Message" class="Str"(error in=w368, "Blinking"=w365, "Visible"=w365) -> (error out=w367:errorcluster)  [unwired: 1 in, 1 out]
            n211 = case shown="Error .." w367 {
              selector: w367 -> [_ w380]
              tunnel: w375 -> [_ w383]
              tunnel: w373 -> [w377 w381]
              tunnel: [w377 w379] -> w374
              tunnel: "Detector Configure. Sending updated FITS files to server." ("Message") -> [w376 _]
              tunnel: [w376 "Error transferring files to Detector Server" ("Message")] -> w363
              frame No Error {
              }
              frame Error {
                n212 = Generate User Event(user event=w383, event data cluster="Error" ("event data")) -> ()  [unwired: 2 in, 2 out]
                n213 = Bundle By Name(cluster=w381, "error"=w380) -> (w379:T15)
              }
            }
            n214 = call "CC SubSystem Message.vi"("Subsystem"="Detector", "Message"=w363) -> ()  [unwired: 9 in, 1 out]
          }
          frame "Shutdown" {
            n215 = Unbundle By Name(w391) -> ("Detector ref"=w390:refnum<class "Detector Class.lvclass">, "Name"=w387:string, "Detector Config"=w389:T7)
            n216 = call "Rd Wr detector settings json.vi"("Detector Name"=w387, "Write? (F:Read)"=TRUE, "Detector Config"=w389) -> ()  [unwired: 7 in, 2 out]
            n217 = call-dynamic "Detector Close.vi"("Detector Class in"=w390) -> ("error out"=w386:errorcluster)  [unwired: 9 in, 1 out]
            n218 = call <vilib>:"Clear Errors.vi"("error in (no error)"=w386) -> ()  [unwired: 5 in, 2 out]
            n219 = call "CC SubSystem Message.vi"("Subsystem"="Detector", "Message"="Detector shutdown.") -> ()  [unwired: 9 in, 1 out]
          }
        }
      }
      event Value Change {
        n220 = event-data() -> ()  [unwired: 1 in, 6 out]
        n221 = case shown="\"Engineering\"" "Mode" {
          tunnel: [bool[] [TRUE, FALSE, FALSE, FALSE, FALSE] bool[] [TRUE, TRUE, TRUE, TRUE, TRUE]] -> w394
          frame "User", Default {
          }
          frame "Engineering" {
          }
        }
        n222 = property on="Tab Control" class="TabCtl (strict)"() -> ("Pages"=w395:refnum<vi>[])  [unwired: 2 in, 2 out]
        n223 = for {
          tunnel: w395 -> [w398] mode=indexing
          tunnel: w394 -> [w397] mode=indexing
          n224 = property class="Page"(reference=w398, "PageVis"=w397) -> ()  [unwired: 1 in, 2 out]
        }
      }
      event "Target Name": Value Change {
        n225 = event-data() -> ()  [unwired: 1 in, 6 out]
        n226 = call "Rd Wr Current Status json.vi"() -> ("Current Status"=w404:T21)  [unwired: 10 in, 1 out]
        n227 = Bundle By Name(cluster=w404, "Target"="Target Name") -> (w402:T21)
        n228 = call "Rd Wr Current Status json.vi"("Write? (F:Read)"=TRUE, "Current Status"=w402) -> ()  [unwired: 8 in, 2 out]
      }
      event "Integration Time", "Frame Integration Time": Value Change {
        n229 = event-data() -> ()  [unwired: 1 in, 6 out]
        n230 = Unbundle By Name(w418) -> ("Detector ref"=w417:refnum<class "Detector Class.lvclass">, "state"=w411:refnum<user-event>)
        n231 = Generate User Event(user event=w411, event data cluster="Set Mode" ("event data")) -> ()  [unwired: 2 in, 2 out]
        n232 = Bundle By Name(cluster=w418, "Detector Config.Integration Mode"="Integration Mode", "Detector Config.Integration Time"="Integration Time", "Detector Config.Frame Int Time"="Frame Integration Time") -> (w408:T15)
        n233 = Quotient & Remainder(x="Integration Time", y="Frame Integration Time") -> (floor(x/y)=→"Number Frames":dbl)  [unwired: 1 out]
        n234 = property on="Integration Time" class="DigNum (strict)"("Minimum"="Frame Integration Time") -> ()  [unwired: 2 in, 2 out]
        n235 = Unbundle By Name(w408) -> ("Detector Config"=w409:T7)
        n236 = Unbundle By Name(w408) -> ("Name"=w407:string)
        n237 = call-dynamic "Write Detector Config.vi"("Detector Config"=w409, "Detector Class in"=w417) -> ("Detector Class out"=w416:refnum<class "Detector Class.lvclass">)  [unwired: 8 in, 1 out]
        n238 = call "Rd Wr detector settings json.vi"("Detector Name"=w407, "Write? (F:Read)"=TRUE, "Detector Config"=w409) -> ()  [unwired: 7 in, 2 out]
        n239 = Bundle By Name(cluster=w408, "Detector ref"=w416) -> (w415:T15)
      }
      event "Clear Log": Value Change {
        n240 = event-data() -> ()  [unwired: 1 in, 6 out]
        n241 = call "lib Quick Message Log.vi"("Clear"=TRUE) -> ("Log"=w420:string)  [unwired: 9 in, 1 out]
        n242 = local write "Messages"(w420) -> ()
      }
      event "Standalone": Value Change {
        n243 = event-data() -> ("NewVal"=w423:bool)  [unwired: 1 in, 5 out]
        n244 = property on="Close" class="Bool"("Visible"=w423) -> ()  [unwired: 2 in, 2 out]
      }
      event "Detector Name": Value Change {
        n245 = event-data() -> ("NewVal"=w430:string)  [unwired: 1 in, 5 out]
        n246 = Unbundle By Name(w428) -> ("Detector ref"=w426:refnum<class "Detector Class.lvclass">, "state"=w427:refnum<user-event>)
        n247 = call-dynamic "Detector Close.vi"("Detector Class in"=w426) -> ()  [unwired: 9 in, 2 out]
        n248 = Generate User Event(user event=w427, event data cluster="init" ("event data")) -> ()  [unwired: 2 in, 2 out]
        n249 = Bundle By Name(cluster=w428, "Name"=w430) -> (w429:T15)
      }
      event "Image List": Value Change {
        n250 = event-data() -> ()  [unwired: 1 in, 6 out]
        n251 = Unbundle By Name(w443) -> ("Images"=w442:T8[])
        n252 = local read "Messages"() -> (w438:string)
        n253 = Index Array(array=w442, index="Image List") -> (element=w440:T8)
        n254 = Unbundle By Name(w440) -> ("FITS file"=w436:path)
        n255 = call "CC FITS Read Image.vi"("FITS File Path"=w436) -> ("error out"=w434:errorcluster, "Image"=w435:sgl[][])  [unwired: 9 in]
        n256 = Select(t="FITS file format is unreadable", s=w434, f="FITS File Opened.") -> (s? t:f=w431:string)
        n257 = local write "image"(w435) -> ()
        n258 = Concatenate Strings(w438, "\r\n", w431) -> (w437:string)
        n259 = local write "Messages"(w437) -> ()
      }
      event "send config": Value Change {
        n260 = event-data() -> ()  [unwired: 1 in, 6 out]
        n261 = Unbundle By Name(w444) -> ("state"=w446:refnum<user-event>)
        n262 = Generate User Event(user event=w446, event data cluster="Send FITS Files" ("event data")) -> ()  [unwired: 2 in, 2 out]
      }
      event "Get Image": Value Change {
        n263 = event-data() -> ()  [unwired: 1 in, 6 out]
        n264 = Unbundle By Name(w449) -> ("state"=w448:refnum<user-event>)
        n265 = Generate User Event(user event=w448, event data cluster="Get Image" ("event data")) -> ()  [unwired: 2 in, 2 out]
      }
      event "Reconnect": Value Change {
        n266 = event-data() -> ()  [unwired: 1 in, 6 out]
        n267 = Unbundle By Name(w453) -> ("state"=w451:refnum<user-event>, "Detector ref"=w452:refnum<class "Detector Class.lvclass">)
        n268 = call-dynamic "Detector Close.vi"("Detector Class in"=w452) -> ()  [unwired: 9 in, 2 out]
        n269 = Generate User Event(user event=w451, event data cluster="connect" ("event data")) -> ()  [unwired: 2 in, 2 out]
      }
      event "Re-init": Value Change {
        n270 = event-data() -> ()  [unwired: 1 in, 6 out]
        n271 = Unbundle By Name(w456) -> ("state"=w455:refnum<user-event>)
        n272 = Generate User Event(user event=w455, event data cluster="init detectors" ("event data")) -> ()  [unwired: 2 in, 2 out]
      }
      event Value Change {
        n273 = event-data() -> ()  [unwired: 1 in, 1 out]
        n274 = Unbundle By Name(w459) -> ("state"=w458:refnum<user-event>)
        n275 = Generate User Event(user event=w458, event data cluster="save" ("event data")) -> ()  [unwired: 2 in, 2 out]
        n276 = Bundle By Name(cluster=w459, "Detector Config.Detector Computer"="Detector Computer") -> (w460:T15)
      }
      event "FITS hdr template0", "FITS hdr template1", "FITS Data File Path": Value Change {
        n277 = event-data() -> ()  [unwired: 1 in, 6 out]
        n278 = Unbundle By Name(w462) -> ("state"=w464:refnum<user-event>)
        n279 = Generate User Event(user event=w464, event data cluster="save" ("event data")) -> ()  [unwired: 2 in, 2 out]
        n280 = Bundle By Name(cluster=w462, "Detector Config.FITS hdr template0"="FITS hdr template0", "Detector Config.FITS hdr template1"="FITS hdr template1", "Detector Config.FITS Data File Path"="FITS Data File Path") -> (w465:T15)
      }
      event "Sim FITS File Path": Value Change {
        n281 = event-data() -> ()  [unwired: 1 in, 6 out]
        n282 = Unbundle By Name(w470) -> ("state"=w472:refnum<user-event>)
        n283 = Generate User Event(user event=w472, event data cluster="save" ("event data")) -> ()  [unwired: 2 in, 2 out]
        n284 = Bundle By Name(cluster=w470, "Detector Config.Sim Folder"="Sim FITS File Path") -> (w473:T15)
      }
      event Value Change {
        n285 = event-data() -> ()  [unwired: 1 in, 6 out]
        n286 = Unbundle By Name(w474) -> ("state"=w476:refnum<user-event>)
        n287 = Generate User Event(user event=w476, event data cluster="save" ("event data")) -> ()  [unwired: 2 in, 2 out]
        n288 = Bundle By Name(cluster=w474, "Detector Config.FITS Detector Settings"="FITS Detector Settings") -> (w477:T15)
      }
      event "Offsets": Value Change {
        n289 = event-data() -> ()  [unwired: 1 in, 6 out]
        n290 = Unbundle By Name(w479) -> ("state"=w481:refnum<user-event>)
        n291 = Generate User Event(user event=w481, event data cluster="save" ("event data")) -> ()  [unwired: 2 in, 2 out]
        n292 = Bundle By Name(cluster=w479, "Detector Config.Offsets"="Offsets") -> (w482:T15)
      }
      event "Close": Value Change {
        n293 = event-data() -> ()  [unwired: 1 in, 2 out]
        n294 = Unbundle By Name(w486) -> ("state"=w485:refnum<user-event>)
        n295 = Generate User Event(user event=w485, event data cluster="Shutdown" ("event data")) -> ()  [unwired: 2 in, 2 out]
      }
    }
  }
